vi "Check If Pixels Belong In Sector Removed FIFO Check.vi"() -> (3 "FIFO Timeout?":bool)   [LabVIEW 2013]
uses:
  FPGA/Sector/Accumulate/Single Sector Pixel Cluster.ctl
  <vilib>/rvi/Emulation/niFpgaSctlEmulationGetInTimedLoop.vi
  FPGA/Globals/Sector Parameter Global.vi
  FPGA/Globals/Pixel Location Global.vi
  <vilib>/rvi/DataTransferAndStorage/Container/Common/niFpgaContainerGetUniqueNameForEmu.vi
  <vilib>/rvi/FIFO/Fifo_Resource/nirvififoEmulationSetSize.vi
  <vilib>/rvi/Emulation/niFpgaSctlEmulationFifoFullMgr.vi
  <vilib>/rvi/errors/niFpgaSetErrorForExecOnDevCompSimple.vi
  <vilib>/rvi/eio/common/nirviEmuReportErrorAndStop.vi
  <vilib>/rvi/Emulation/niFpgaSctlEmulationResourceMgr.vi
  <vilib>/rvi/DataTransferAndStorage/Container/XNode/niFpgaContainer.xnode
  <vilib>/rvi/FIFO/Fifo_Resource/nirvififoEmulationRead.vi
  <vilib>/rvi/FIFO/Fifo_Resource/nirvififoEmulationWrite.vi
  FPGA/FPGA Image Processing.lvlib
panel:
  out "End of  Data?":bool
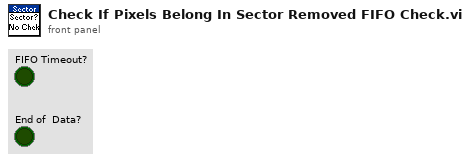
[diagram p1: front panel]
types:
  T1 = typedef "Sector Parameter Cluster.ctl" = cluster{"Start Angle":fxp<+/-,17,2>, "End Angle":fxp<+,17,3>, "Inner Radius":u16, "Outter Radius":u16, "Hinge X":u16, "Hinge Y":u16, "NumWingSectors":u8}
  T2 = typedef "Single Sector Pixel Cluster.ctl" = cluster{"Sector #":u8, "Pixel Value":u8}
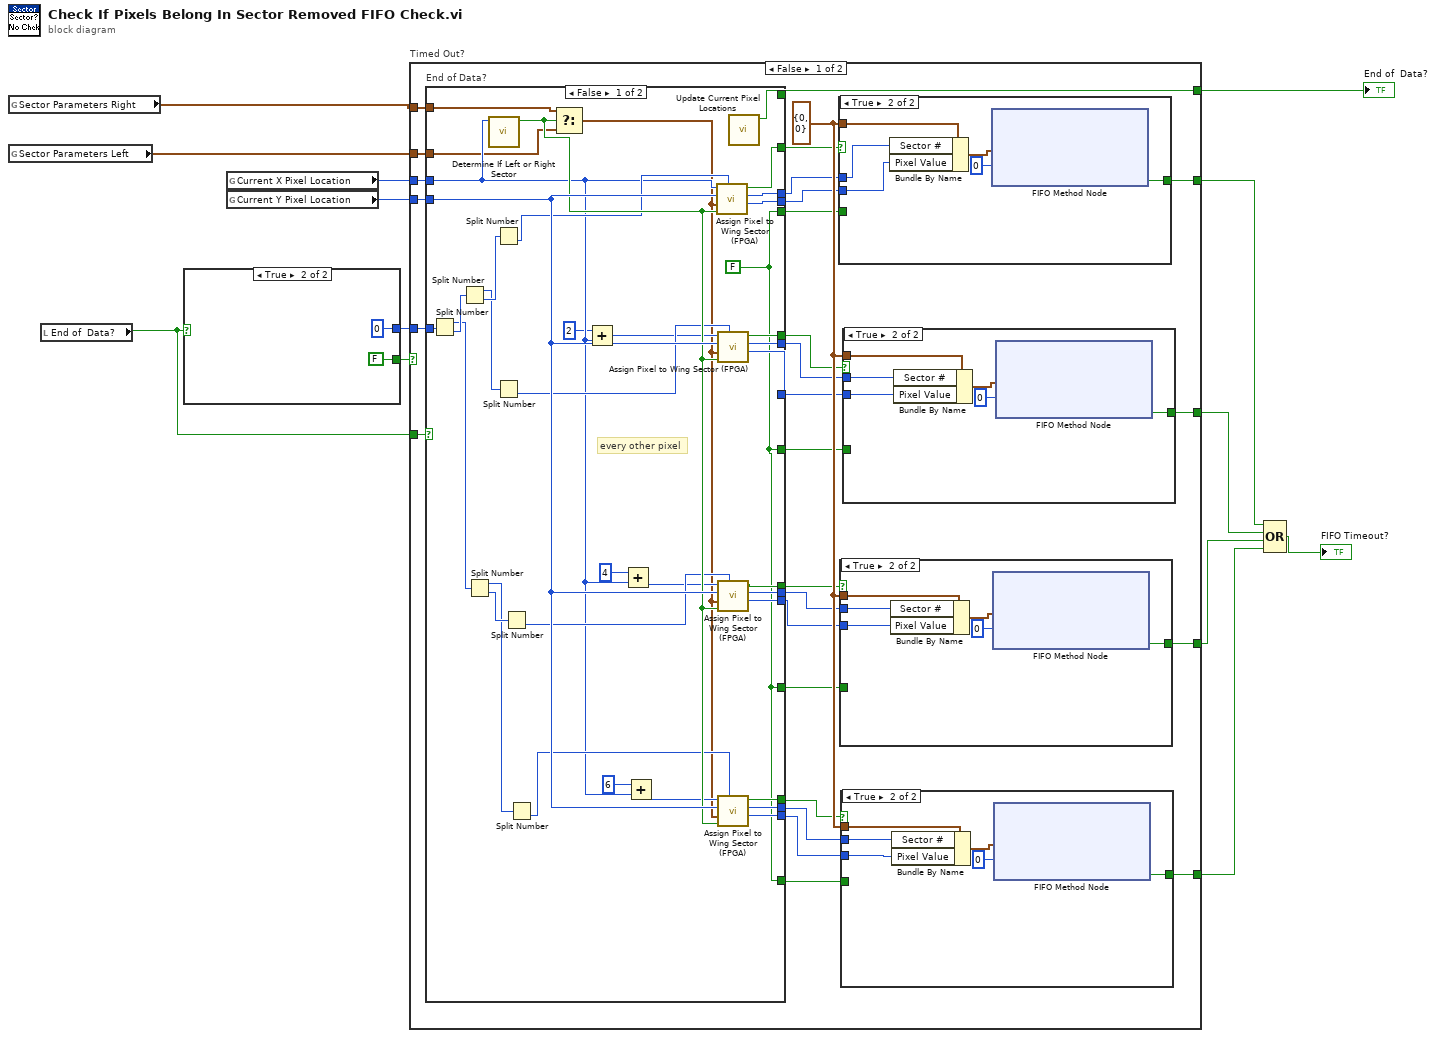
[diagram p0: block diagram]
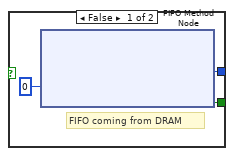
[diagram p2: hidden frame]
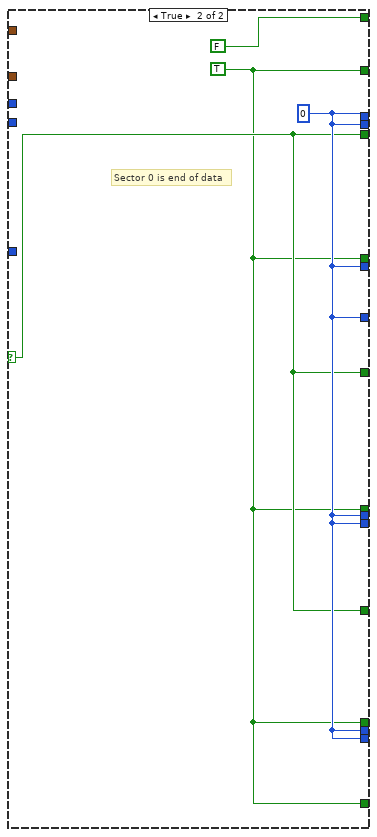
[diagram p3: hidden frame]
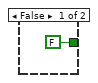
[diagram p4: hidden frame]
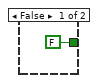
[diagram p5: hidden frame]
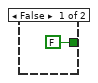
[diagram p6: hidden frame]
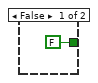
[diagram p7: hidden frame]
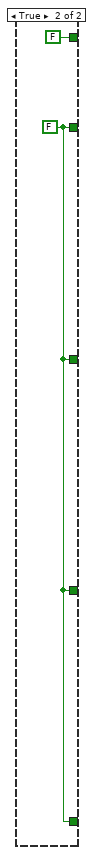
[diagram p8: hidden frame]
diagram:
  n1 = global read "Sector Parameter Global.vi" "Sector Parameters Right"() -> (w10:T1)
  n2 = global read "Sector Parameter Global.vi" "Sector Parameters Left"() -> (w9:T1)
  n3 = local read "End of  Data?"() -> (w11:bool)
  n4 = case shown="True" w11 {
    tunnel: [w15 FALSE ("Timed Out?")] -> w8
    tunnel: [w14 u64 0 ("Element")] -> w5
    frame False {
      # "FIFO coming from DRAM"
      n5 = xnode ("FIFO Method Node")("Timeout"=0) -> ("Element"=w14:u64, "Timed Out?"=w15:bool)  [unwired: 1 in, 1 out]
    }
    frame True {
    }
  }
  n6 = global read "Pixel Location Global.vi" "Current X Pixel Location"() -> (w7:u16)
  n7 = global read "Pixel Location Global.vi" "Current Y Pixel Location"() -> (w6:u16)
  n8 = case "Timed Out?" shown="False" w8 {
    tunnel: w7 -> [w37 _]
    tunnel: w6 -> [w46 _]
    tunnel: w5 -> [w44 _]
    tunnel: [w45 w117] -> w4
    tunnel: [w43 w117] -> w3
    tunnel: [w42 w117] -> w2
    tunnel: [w40 w117] -> w1
    tunnel: w10 -> [w39 _]
    tunnel: w9 -> [w38 _]
    tunnel: [w24 FALSE ("End of Average Data?")] -> w13
    tunnel: w11 -> [w23 _]
    frame False {
      w41 = T2 {"Sector #"=0, "Pixel Value"=0} ("Single Sector Pixel")
      n9 = case "End of Data?" shown="False" w23 {
        selector: w23 -> [_ w85]
        tunnel: w46 -> [w83 _]
        tunnel: w44 -> [w79 _]
        tunnel: w39 -> [w49 _]
        tunnel: w38 -> [w48 _]
        tunnel: w37 -> [w57 _]
        tunnel: [w73 w84] -> w36
        tunnel: [w72 w86] -> w35
        tunnel: [w71 w86] -> w34
        tunnel: [w70 w84] -> w33
        tunnel: [w69 w86] -> w32
        tunnel: [w67 w86] -> w31
        tunnel: [w66 w84] -> w30
        tunnel: [w65 w86] -> w29
        tunnel: [w63 w86] -> w28
        tunnel: [w62 w84] -> w27
        tunnel: [w61 w86] -> w26
        tunnel: [w60 w86] -> w25
        tunnel: [w58 FALSE ("End of data?")] -> w24
        tunnel: [w56 w85] -> w22
        tunnel: [w56 w85] -> w21
        tunnel: [w56 w85] -> w20
        tunnel: [w56 w84] -> w19
        frame False {
          w56 = FALSE
          # "every other pixel"
          n10 = Split Number(x=w79) -> (hi(x)=w81:u32, lo(x)=w82:u32)
          n11 = Split Number(x=w82) -> (hi(x)=w78:u16, lo(x)=w80:u16)
          n12 = Split Number(x=w81) -> (hi(x)=w76:u16, lo(x)=w77:u16)
          n13 = call "Determine If Left or Right Sector.vi"("X Pixel Location"=w57) -> ("Right Sector?"=w75:bool)  [unwired: 10 in]
          n14 = Split Number(x=w80) -> (lo(x)=w74:u8)  [unwired: 1 out]
          n15 = Split Number(x=w78) -> (lo(x)=w68:u8)  [unwired: 1 out]
          n16 = Split Number(x=w77) -> (lo(x)=w64:u8)  [unwired: 1 out]
          n17 = Split Number(x=w76) -> (lo(x)=w59:u8)  [unwired: 1 out]
          n18 = Select(t=w49, s=w75, f=w48) -> (s? t:f=w47:T1)
          n19 = Add(x=u16 2, y=w57) -> (x+y=w52:u16)
          n20 = Add(x=u16 4, y=w57) -> (x+y=w51:u16)
          n21 = Add(x=u16 6, y=w57) -> (x+y=w50:u16)
          n22 = call "Assign Pixel to Wing Sector (FPGA).vi"("Pixel Intensity In"=w74, "Right Wing?"=w75, "Sector Parameters"=w47, "Pixel Y"=w83, "Pixel X"=w57) -> ("Pixel Intensity Out"=w71:u8, "sector #"=w72:u8, "output valid"=w73:bool)  [unwired: 3 in]
          n23 = call "Assign Pixel to Wing Sector (FPGA).vi"("Pixel Intensity In"=w68, "Right Wing?"=w75, "Sector Parameters"=w47, "Pixel Y"=w83, "Pixel X"=w52) -> ("Pixel Intensity Out"=w67:u8, "sector #"=w69:u8, "output valid"=w70:bool)  [unwired: 3 in]
          n24 = call "Assign Pixel to Wing Sector (FPGA).vi"("Pixel Intensity In"=w64, "Right Wing?"=w75, "Sector Parameters"=w47, "Pixel Y"=w83, "Pixel X"=w51) -> ("Pixel Intensity Out"=w63:u8, "sector #"=w65:u8, "output valid"=w66:bool)  [unwired: 3 in]
          n25 = call "Assign Pixel to Wing Sector (FPGA).vi"("Pixel Intensity In"=w59, "Right Wing?"=w75, "Sector Parameters"=w47, "Pixel Y"=w83, "Pixel X"=w50) -> ("Pixel Intensity Out"=w60:u8, "sector #"=w61:u8, "output valid"=w62:bool)  [unwired: 3 in]
          n26 = call "Update Current Pixel Locations.vi"() -> ("End of data?"=w58:bool)  [unwired: 11 in]
        }
        frame True {
          w86 = u8 0 ("sector #")
          w84 = TRUE ("output valid")
          # "Sector 0 is end of data"
        }
      }
      n27 = case shown="True" w36 {
        tunnel: w41 -> [_ w110]
        tunnel: [FALSE ("Timed Out?") w113] -> w45
        tunnel: w35 -> [_ w111]
        tunnel: w34 -> [_ w112]
        tunnel: w22 -> [_ _]
        frame False {
        }
        frame True {
          n28 = Bundle By Name(cluster=w110, "Sector #"=w111, "Pixel Value"=w112) -> (w114:T2)
          n29 = xnode ("FIFO Method Node")("Element"=w114, "Timeout"=0) -> ("Timed Out?"=w113:bool)  [unwired: 1 in, 1 out]
        }
      }
      n30 = case shown="True" w30 {
        tunnel: w41 -> [_ w101]
        tunnel: [FALSE ("Timed Out?") w98] -> w42
        tunnel: w29 -> [_ w96]
        tunnel: w28 -> [_ w97]
        tunnel: w20 -> [_ _]
        frame False {
        }
        frame True {
          n31 = Bundle By Name(cluster=w101, "Sector #"=w96, "Pixel Value"=w97) -> (w99:T2)
          n32 = xnode ("FIFO Method Node")("Element"=w99, "Timeout"=0) -> ("Timed Out?"=w98:bool)  [unwired: 1 in, 1 out]
        }
      }
      n33 = case shown="True" w27 {
        tunnel: w41 -> [_ w94]
        tunnel: [FALSE ("Timed Out?") w91] -> w40
        tunnel: w26 -> [_ w89]
        tunnel: w25 -> [_ w90]
        tunnel: w19 -> [_ _]
        frame False {
        }
        frame True {
          n34 = Bundle By Name(cluster=w94, "Sector #"=w89, "Pixel Value"=w90) -> (w92:T2)
          n35 = xnode ("FIFO Method Node")("Element"=w92, "Timeout"=0) -> ("Timed Out?"=w91:bool)  [unwired: 1 in, 1 out]
        }
      }
      n36 = case shown="True" w33 {
        tunnel: w41 -> [_ w108]
        tunnel: [FALSE ("Timed Out?") w105] -> w43
        tunnel: w32 -> [_ w103]
        tunnel: w31 -> [_ w104]
        tunnel: w21 -> [_ _]
        frame False {
        }
        frame True {
          n37 = Bundle By Name(cluster=w108, "Sector #"=w103, "Pixel Value"=w104) -> (w106:T2)
          n38 = xnode ("FIFO Method Node")("Element"=w106, "Timeout"=0) -> ("Timed Out?"=w105:bool)  [unwired: 1 in, 1 out]
        }
      }
    }
    frame True {
      w117 = FALSE ("Timed Out?")
    }
  }
  "End of  Data?" <- w13
  n39 = Compound Arithmetic op=OR(w4, w3, w2, w1) -> (→"FIFO Timeout?":bool)
